vi "PH_Beamline_Common.set Mirror.vi"(0 "Alignment (left down to right up)":T3=enum."left down to right up", 1 "Size (36x36)":T2, 2 "CtlRef":refnum<vi>, 3 "Status (on/true/in)":T1=2 items=["no info", "off/false/out", "on/true/in", "Failure", "Alarm", "Status 1", "Status 2", "Status 3"], 4 "GUI Instance does not exist or here?":bool, 5 "error in (no error)":errorcluster, 6 "Visible (true)":bool=TRUE, 7 "Tip Strip (N/A)":string="N/A") -> (19 "error out":errorcluster)   [LabVIEW 2014, in "PH_Beamline_Common.lvlib"]
uses:
  PH_Beamline_Common.lvlib
  PH_Common/Picture/PH_Picture.Alignment.ctl
  PH_Common/Picture/PH_Picture.Size.ctl
  PH_StatusHandler/PH_StatusHandler.Status.ctl
  PH_Common/PH_Common.lvlib
  PH_StatusHandler/PH_StatusHandler.lvlib
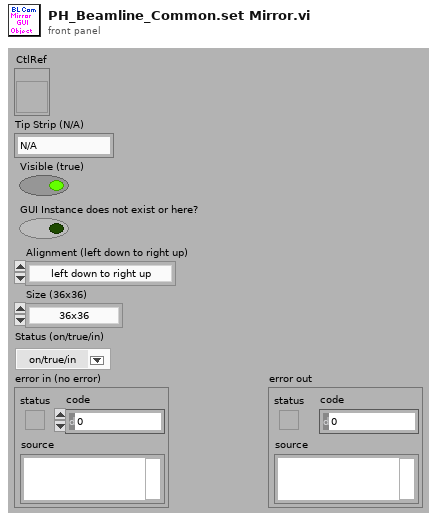
[diagram p1: front panel]
types:
  T1 = typedef "PH_StatusHandler.lvlib/PH_StatusHandler.Status.ctl" = i16
  T2 = typedef "PH_Common.lvlib/PH_Picture.Size.ctl" = enum16{"36x36", "48x48", "24x36", "36x24", "12x60", "60x12"}
  T3 = typedef "PH_Common.lvlib/PH_Picture.Alignment.ctl" = enum16{"neutral", "left", "right", "up", "down", "vertical", "horizontal", "left down to right up", "left up to right down"}
  T4 = cluster{"left":i16, "top":i16, "right":i16, "bottom":i16}
  T5 = cluster{"Width":u16, "Style":enum32{"Solid", "Dash", "Dot", "DashDot", "DashDotDot"}}
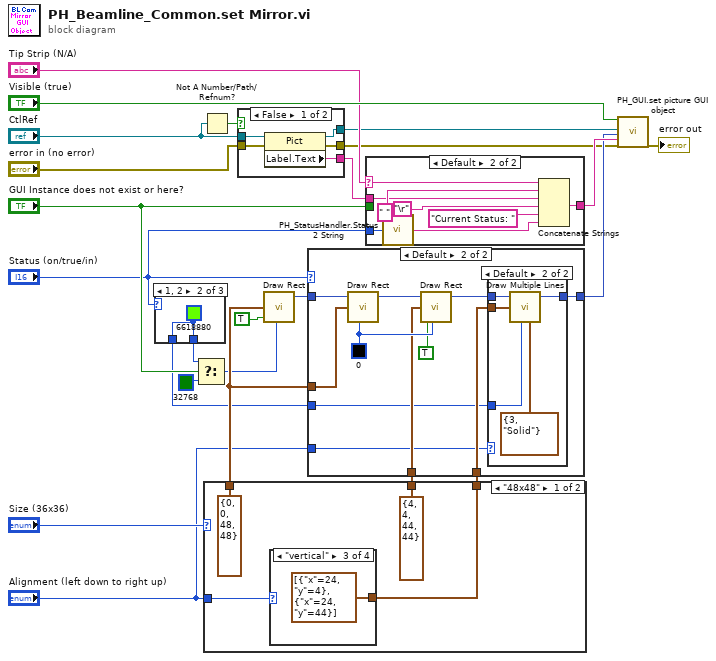
[diagram p0: block diagram]
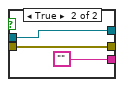
[diagram p2: hidden frame]
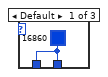
[diagram p5: hidden frame]
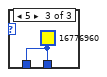
[diagram p6: hidden frame]
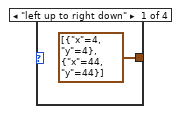
[diagram p7: hidden frame]
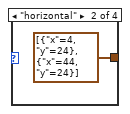
[diagram p8: hidden frame]
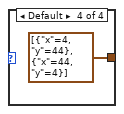
[diagram p9: hidden frame]
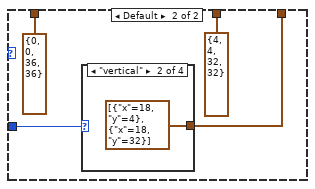
[diagram p10: hidden frame]
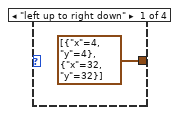
[diagram p11: hidden frame]
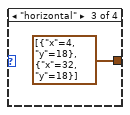
[diagram p12: hidden frame]
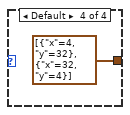
[diagram p13: hidden frame]
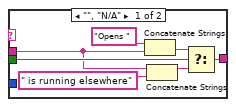
[diagram p14: hidden frame]
diagram:
  n1 = case shown="1, 2" "Status (on/true/in)" {
    tunnel: [w25 w26 w27] -> w12
    tunnel: [w25 w26 w27] -> w11
    frame Default {
      w25 = u32 16860
    }
    frame 1, 2 {
      w26 = u32 6618880
    }
    frame 5 {
      w27 = u32 16776960
    }
  }
  n2 = Select(t=w12, s="GUI Instance does not exist or here?", f=u32 32768 ("Color Box")) -> (s? t:f=w13:u32)
  n3 = Not A Number/Path/Refnum?(number/path/refnum="CtlRef") -> (NaN/Path/Refnum?=w8:bool)
  n4 = case shown="\"48x48\"" "Size (36x36)" {
    tunnel: [T4 {"left"=0, "top"=0, "right"=48, "bottom"=48} ("rect") T4 {"left"=0, "top"=0, "right"=36, "bottom"=36} ("rect")] -> w17
    tunnel: [T4 {"left"=4, "top"=4, "right"=44, "bottom"=44} ("rect") T4 {"left"=4, "top"=4, "right"=32, "bottom"=32} ("rect")] -> w15
    tunnel: [w29 w37] -> w14
    tunnel: "Alignment (left down to right up)" -> [w28 w36]
    frame "48x48" {
      n5 = case shown="\"vertical\"" w28 {
        tunnel: [cluster{"x":i16, "y":i16}[] [{"x"=4, "y"=4}, {"x"=44, "y"=44}] ("line endpoints") cluster{"x":i16, "y":i16}[] [{"x"=4, "y"=24}, {"x"=44, "y"=24}] ("line endpoints") cluster{"x":i16, "y":i16}[] [{"x"=24, "y"=4}, {"x"=24, "y"=44}] ("line endpoints") cluster{"x":i16, "y":i16}[] [{"x"=4, "y"=44}, {"x"=44, "y"=4}] ("line endpoints")] -> w29
        frame "left up to right down" {
        }
        frame "horizontal" {
        }
        frame "vertical" {
        }
        frame Default {
        }
      }
    }
    frame Default {
      n6 = case shown="\"vertical\"" w36 {
        tunnel: [cluster{"x":i16, "y":i16}[] [{"x"=4, "y"=4}, {"x"=32, "y"=32}] ("line endpoints") cluster{"x":i16, "y":i16}[] [{"x"=18, "y"=4}, {"x"=18, "y"=32}] ("line endpoints") cluster{"x":i16, "y":i16}[] [{"x"=4, "y"=18}, {"x"=32, "y"=18}] ("line endpoints") cluster{"x":i16, "y":i16}[] [{"x"=4, "y"=32}, {"x"=32, "y"=4}] ("line endpoints")] -> w37
        frame "left up to right down" {
        }
        frame "vertical" {
        }
        frame "horizontal" {
        }
        frame Default {
        }
      }
    }
  }
  n7 = case shown="False" w8 {
    tunnel: "CtlRef" -> [w48 w51]
    tunnel: "error in (no error)" -> [w47 w50]
    tunnel: [w46 w51] -> w4
    tunnel: [w45 w50] -> w3
    tunnel: [w44 ""] -> w2
    frame False {
      n8 = property class="Pict"(reference=w48, error in=w47) -> (reference out=w46:refnum<vi>, error out=w45:errorcluster, "Label.Text"=w44:string)
    }
    frame True {
    }
  }
  n9 = call <vilib>:"Draw Rect.vi"("rect"=w17, "fill?(F)"=TRUE, "color(black)"=w13) -> ("new picture"=w18:picture)  [unwired: 6 in]
  n10 = case shown="Default" "Status (on/true/in)" {
    tunnel: w18 -> [w52 w63]
    tunnel: w17 -> [_ w62]
    tunnel: [w52 w60] -> w16
    tunnel: w15 -> [_ w58]
    tunnel: w14 -> [_ w57]
    tunnel: w11 -> [_ w56]
    tunnel: "Alignment (left down to right up)" -> [_ w53]
    frame 1 {
    }
    frame Default {
      w59 = u32 0
      n11 = call <vilib>:"Draw Rect.vi"("picture"=w63, "rect"=w62, "color(black)"=w59) -> ("new picture"=w61:picture)  [unwired: 6 in]
      n12 = call <vilib>:"Draw Rect.vi"("picture"=w61, "rect"=w58, "fill?(F)"=TRUE, "color(black)"=w59) -> ("new picture"=w55:picture)  [unwired: 5 in]
      n13 = case shown="Default" w53 {
        tunnel: [w64 w69] -> w60
        tunnel: w57 -> [_ w68]
        tunnel: w56 -> [_ w67]
        tunnel: w55 -> [w64 w66]
        frame "neutral" {
        }
        frame Default {
          n14 = call <vilib>:"Draw Multiple Lines.vi"("picture"=w66, "line endpoints"=w68, "color(black)"=w67, "pen"=T5 {"Width"=3, "Style"=enum."Solid"}) -> ("new picture"=w69:picture)  [unwired: 5 in]
        }
      }
    }
  }
  n15 = case shown="Default" "Tip Strip (N/A)" {
    selector: "Tip Strip (N/A)" -> [_ w84]
    tunnel: [w73 w81] -> w23
    tunnel: "GUI Instance does not exist or here?" -> [w75 _]
    tunnel: w2 -> [w70 w82]
    tunnel: "Status (on/true/in)" -> [_ w78]
    frame "", "N/A" {
      n16 = Concatenate Strings("Opens " ("string"), w70) -> (w74:string)
      n17 = Concatenate Strings(w70, " is running elsewhere" ("string")) -> (w71:string)
      n18 = Select(t=w74, s=w75, f=w71) -> (s? t:f=w73:string)
    }
    frame Default {
      n19 = call "PH_StatusHandler.Status 2 String.vi"("Status"=w78) -> ("Status as string"=w77:string)
      n20 = Concatenate Strings(w84, " " ("string"), w82, "\r", "Current Status: " ("string"), w77) -> (w81:string)
    }
  }
  n21 = call "PH_GUI.set picture GUI object.vi"("Visible (true)"="Visible (true)", "CtlRef"=w4, "Picture"=w16, "Tip Strip (\"\")"=w23, "error in (no error)"=w3) -> ("error out"=→"error out":errorcluster)  [unwired: 14 in]
